vi "define columns.vi"(10 "Enum Array":refnum<vi>[](array[refnum])) -> (2 "Column Definition":T1[](array[typedef]) {"MinWidth" min=2 step=1; "AutoSizeMode" items=["None"=1, "ColumnHeader"=2, "AllCellsExceptHeader"=4, "AllCells"=6, "DisplayedCellsExceptHeader"=8, "DisplayedCells"=10, "Fill"=16]; "FillWeight" min=1 max=100})   [LabVIEW 2013, in "Table Test Editor Node.lvclass"]
uses:
  Table Test Editor Node.lvclass
  Column/Column Descriptor.ctl
  Column/Column Type.ctl
  <vilib>/NI/Tag Bus/tag/Data Type.ctl
  Table Manager/Call Back Ref Type Def.ctl
  <vilib>/NI/DCAF/Tag Editor Core/Configuration Editor/Classes/Engine Parent/Engine Parent Editor Node.lvclass
  <vilib>/NI/DCAF/Tag Editor Core/Configuration Editor/Classes/Module editor node/module editor node.lvclass
  Column/Column.lvclass
  <vilib>/NI/Tag Bus/tag/tag descriptor.lvclass
  Table Manager/Table Manager.lvclass
  Mapping Column/Mapping Column.lvclass
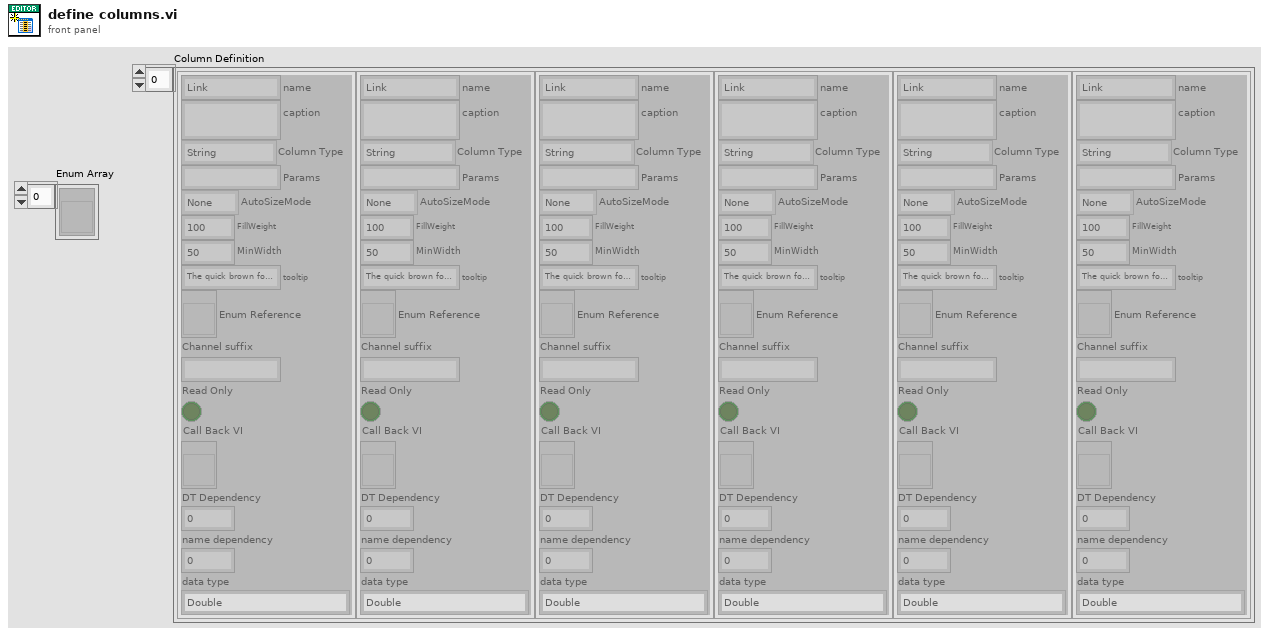
[diagram p1: front panel]
types:
  T1 = typedef "Table Manager.lvlib/Column.lvclass/Column Descriptor.ctl" = cluster{"name":string, "caption":string, "Column Type":T2, "Params":string, "AutoSizeMode":i32, "FillWeight":sgl, "MinWidth":u32, "tooltip":string, "Enum Reference":refnum<vi>, "Channel suffix":string, "Read Only":bool, "Call Back VI":T3, "DT Dependency":i32, "name dependency":i32, "data type":T4}
  T2 = typedef "Table Manager.lvlib/Column.lvclass/Column Type.ctl" = enum16{"String", "Mapping", "Channel Name", "Tag", "Enum", "Data Type", "Numeric"}
  T3 = typedef "Table Manager.lvlib/Table Manager.lvclass/Call Back Ref Type Def.ctl" = refnum<vi>
  T4 = typedef "tag bus.lvlib/tag descriptor.lvclass/Data Type.ctl" = enum16{"Double", "Single", "I64", "I32", "I16", "I8", "U64", "U32", "U16", "U8", "Boolean", "String", "Array of Double", "Array of Single", "Array of I64", "Array of I32", "Array of I16", "Array of I8", "Array of U64", "Array of U32", "Array of U16", "Array of U8", "Array of Boolean", "Array of String"}
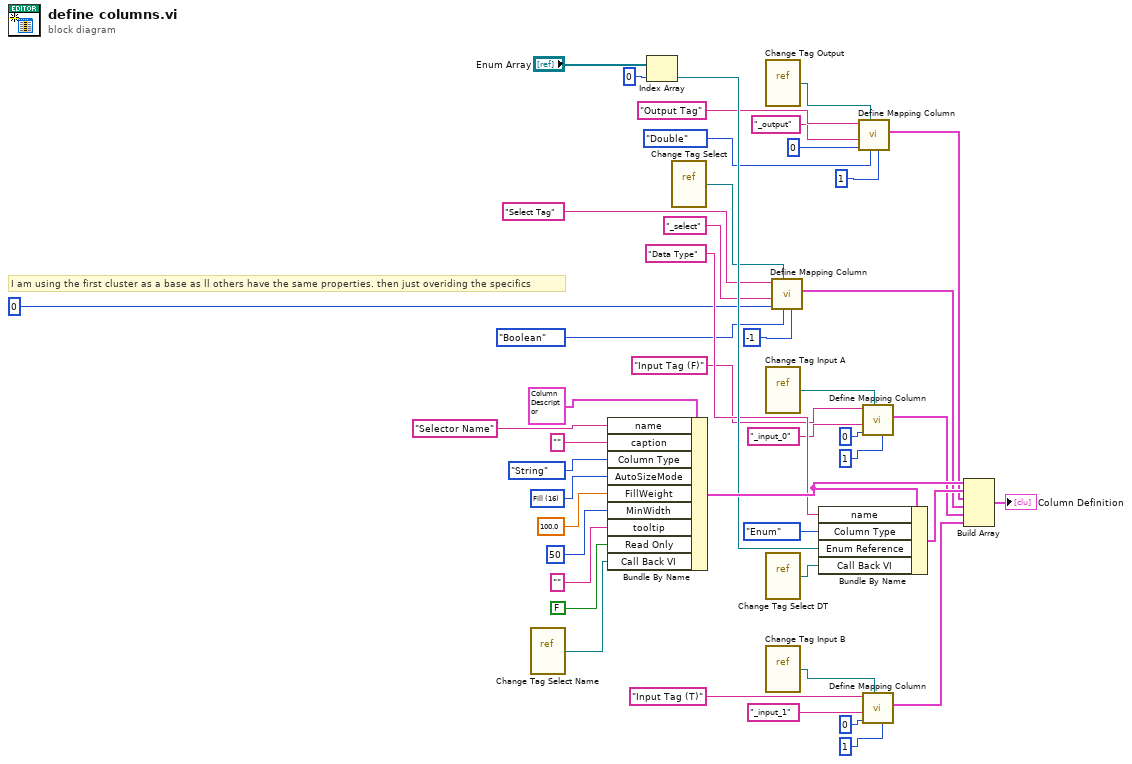
[diagram p0: block diagram]
diagram:
  w33 = 16 items=["None"=1, "ColumnHeader"=2, "AllCellsExceptHeader"=4, "AllCells"=6, "DisplayedCellsExceptHeader"=8, "DisplayedCells"=10, "Fill"=16] ("AutoSizeMode")
  # "I am using the first cluster as a base as ll others have the same properties. then just overiding the specifics"
  n1 = vi-ref "Change Tag Select Name.vi"() -> (w29:refnum<vi>)
  n2 = Bundle By Name(cluster=T1 {"name"="", "caption"="", "Column Type"=enum."String", "Params"="", "AutoSizeMode"=0, "FillWeight"=0.0, "MinWidth"=0, "tooltip"="", "Enum Reference"=refnum, "Channel suffix"="", "Read Only"=FALSE, "Call Back VI"=refnum, "DT Dependency"=0, "name dependency"=0, "data type"=enum."Double"} ("Table Manager.lvlib:Column.lvclass:Column Descriptor"), "name"="Selector Name", "caption"="", "Column Type"=Column_Type."String", "AutoSizeMode"=w33, "FillWeight"=sgl 100.0, "MinWidth"=u32 50, "tooltip"="", "Read Only"=FALSE, "Call Back VI"=w29) -> (w42:T1)
  n3 = Index Array(array="Enum Array", index=0) -> (element=w40:refnum<vi>)
  n4 = vi-ref "Change Tag Select.vi"() -> (w25:refnum<vi>)
  n5 = vi-ref "Change Tag Output.vi"() -> (w24:refnum<vi>)
  n6 = vi-ref "Change Tag Input A.vi"() -> (w26:refnum<vi>)
  n7 = vi-ref "Change Tag Select DT.vi"() -> (w30:refnum<vi>)
  n8 = vi-ref "Change Tag Input B.vi"() -> (w27:refnum<vi>)
  n9 = call "Define Mapping Column.vi"("DT Dependency"=-1, "data type"=Data_Type."Boolean", "Call Back VI"=w25, "name dependency"=0, "Channel suffix"="_select" ("string"), "name"="Select Tag") -> ("Table Manager.lvlib:Column.lvclass:Column Descriptor"=w13:T1)  [unwired: 5 in]
  n10 = Bundle By Name(cluster=w42, "name"="Data Type", "Column Type"=Column_Type."Enum", "Enum Reference"=w40, "Call Back VI"=w30) -> (w45:T1)
  n11 = call "Define Mapping Column.vi"("DT Dependency"=1, "data type"=Data_Type."Double", "Call Back VI"=w24, "name dependency"=0, "Channel suffix"="_output" ("string"), "name"="Output Tag") -> ("Table Manager.lvlib:Column.lvclass:Column Descriptor"=w23:T1)  [unwired: 5 in]
  n12 = call "Define Mapping Column.vi"("DT Dependency"=1, "Call Back VI"=w26, "name dependency"=0, "Channel suffix"="_input_0" ("string"), "name"="Input Tag (F)") -> ("Table Manager.lvlib:Column.lvclass:Column Descriptor"=w3:T1)  [unwired: 6 in]
  n13 = call "Define Mapping Column.vi"("DT Dependency"=1, "Call Back VI"=w27, "name dependency"=0, "Channel suffix"="_input_1" ("string"), "name"="Input Tag (T)") -> ("Table Manager.lvlib:Column.lvclass:Column Descriptor"=w14:T1)  [unwired: 6 in]
  n14 = Build Array(w42, w45, w23, w13, w3, w14) -> (→"Column Definition":T1[])
